vi "Rename Object.vi"(6 "Post Object File Path":path, 8 "error in":errorcluster, 9 "Pre Object File Path":path, 10 "Active Project":refnum<vi>) -> (0 "error out":errorcluster, 2 "Object Ref":refnum<vi>)   [LabVIEW 2025, in "_Rename.lvlib" / "_Rename.lvclass"]
uses:
  _Rename.lvclass
  _Rename.lvclass/_Rename.ctl
  <vilib>/Utility/EditLVLibs/Edit LVLibs.lvlib
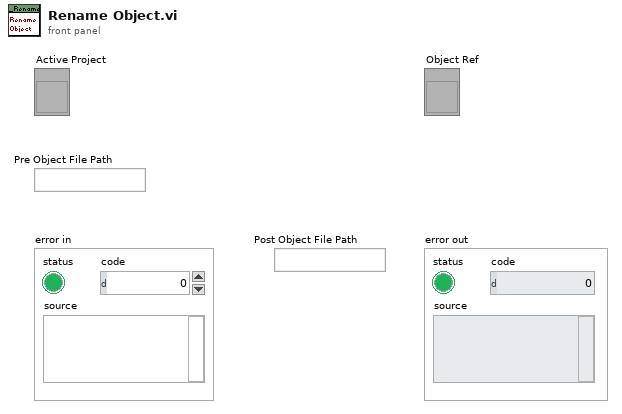
[diagram p1: front panel]
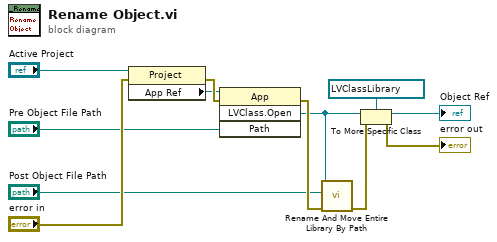
[diagram p0: block diagram]
diagram:
  n1 = property class="Project"(reference="Active Project", error in="error in") -> (error out=w11:errorcluster, "App Ref"=w10:refnum<vi>)  [unwired: 1 out]
  n2 = invoke class="App" method="LVClass.Open"(reference=w10, error in=w11, "Path"="Pre Object File Path") -> (error out=w12:errorcluster, "LVClass.Open"=w8:refnum<vi>)  [unwired: 1 in, 2 out]
  n3 = call <vilib>:"Rename And Move Entire Library By Path.vi"("error in (no error)"=w12, "New library path"="Post Object File Path", "Library ref in"=w8) -> ("error out"=w7:errorcluster)  [unwired: 7 in, 1 out]
  n4 = To More Specific Class(target class=refnum<vi> refnum ("Class in"), reference=w8, error in=w7) -> (specific class reference=→"Object Ref":refnum<vi>, error out=→"error out":errorcluster)
